vi "get_pixel_times.vi"(8 "error in (no error)":errorcluster, 11 "TrajectoryMG100122AODFrameScan in":refnum<class "TrajectoryMH100122AODRAPS.lvclass">) -> (0 "error out":errorcluster, 1 "equilibration time":dbl[unit], 2 "acquisition time":dbl[unit], 3 "TrajectoryMG100122AODFrameScan out":refnum<class "TrajectoryMH100122AODRAPS.lvclass">, 4 "total pixel time":dbl[unit])   [LabVIEW 2010, in "TrajectoryMH100122AODRAPS.lvclass"]
uses:
  TrajectoryMH100122AODRAPS.lvclass
  FPGAWrapper/FPGAWrapperMH120124AOD/FPGAWrapperMH120124RAPS_PXI7813R/FPGAWrapperMH120124RAPS_PXI7813R.lvclass
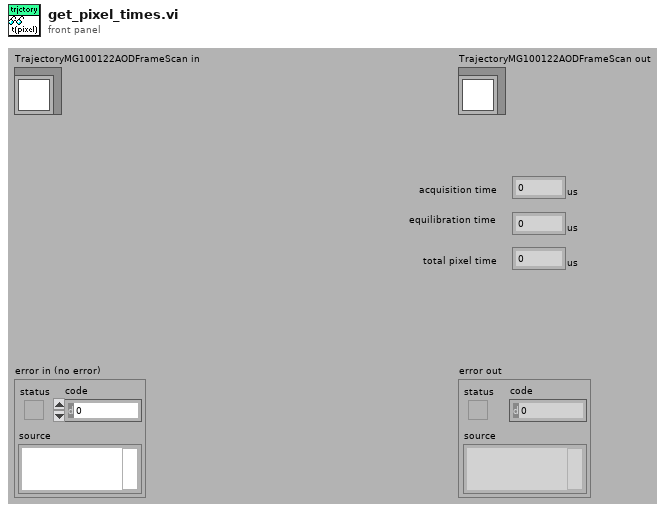
[diagram p1: front panel]
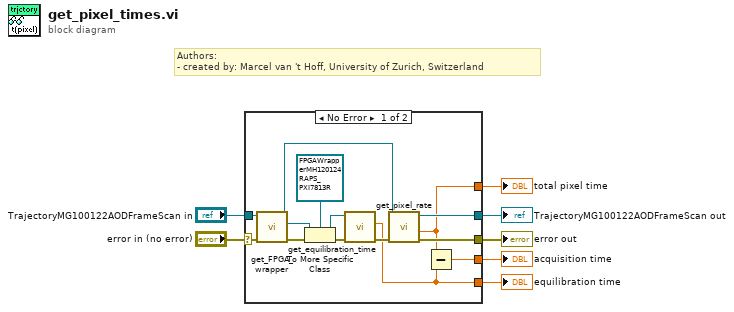
[diagram p0: block diagram]
diagram:
  # "Authors: \n- created by: Marcel van 't Hoff, University of Zurich, Switzerland"
  n1 = case shown="No Error" "error in (no error)" {
    selector: "error in (no error)" -> [w10 w22]
    tunnel: [w21 w22] -> w6
    tunnel: [w20 w23] -> w4
    tunnel: "TrajectoryMG100122AODFrameScan in" -> [w12 w23]
    tunnel: [w8 _] -> w3
    tunnel: [w19 _] -> w2
    tunnel: [w18 _] -> w1
    frame No Error {
      n2 = call-dynamic "get_FPGA_wrapper.vi"("error in (no error)"=w10, "TrajectoryMG100122GenericFPGA in"=w12) -> ("error out"=w17:errorcluster, "GenericFPGAWrapper.lvclass"=w13:refnum<class "GenericFPGAWrapper.lvclass">, "TrajectoryMG100122GenericFPGA out"=w11:refnum<class "TrajectoryMH100122AODRAPS.lvclass">)  [unwired: 7 in]
      n3 = To More Specific Class(target class=refnum<class "FPGAWrapperMH120124RAPS_PXI7813R.lvclass"> refnum ("FPGAWrapperMH120124RAPS_PXI7813R.lvclass"), reference=w13, error in=w17) -> (specific class reference=w15:refnum<class "FPGAWrapperMH120124RAPS_PXI7813R.lvclass">, error out=w16:errorcluster)
      n4 = call-dynamic "get_equilibration_time.vi"("error in (no error)"=w16, "FPGAWrapperMH120124RAPS_PXI7813R in"=w15) -> ("error out"=w9:errorcluster, "AOD equilibration time"=w8:dbl[unit])  [unwired: 7 in, 1 out]
      n5 = call-dynamic "get_pixel_rate.vi"("error in (no error)"=w9, "GenericTrajectory in"=w11) -> ("error out"=w21:errorcluster, "pixel dwell time"=w19:dbl[unit], "GenericTrajectory out"=w20:refnum<class "TrajectoryMH100122AODRAPS.lvclass">)  [unwired: 6 in, 1 out]
      n6 = Subtract(x=w19, y=w8) -> (x-y=w18:dbl[unit])
    }
    frame Error {
    }
  }
  "error out" <- w6
  "TrajectoryMG100122AODFrameScan out" <- w4
  "acquisition time" <- w1
  "equilibration time" <- w3
  "total pixel time" <- w2
